vi "TCPPacket Write Body.vi"(8 "error in (no error)":errorcluster, 11 "JSONPacket in":refnum<class "JSONPacket.lvclass">) -> (0 "error out":errorcluster, 2 "Data":u8[](array[numeric]), 3 "JSONPacket out":refnum<class "JSONPacket.lvclass">)   [LabVIEW 2019, in "JSONPacket.lvclass"]
uses:
  JSONPacket.lvclass
  JSONPacket.lvclass/JSONPacket.ctl
  TCPPacket/TCPPacket.lvclass
  <vilib>/addons/Tools/Unicode/UTF8 Tools.lvlib
  6540c986-0add-4175-90d9-41b83a32c240.vi
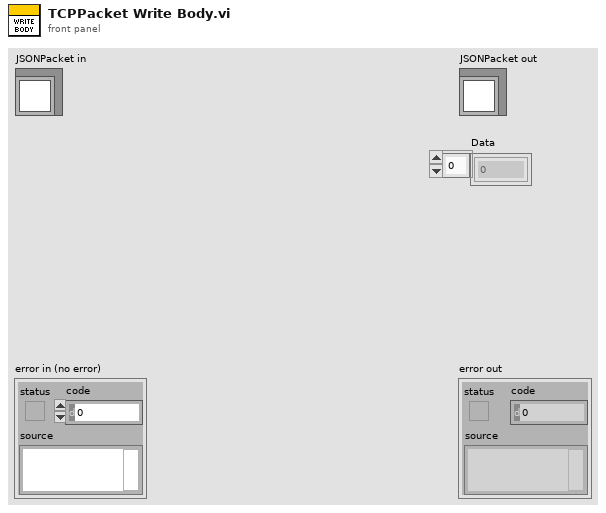
[diagram p1: front panel]
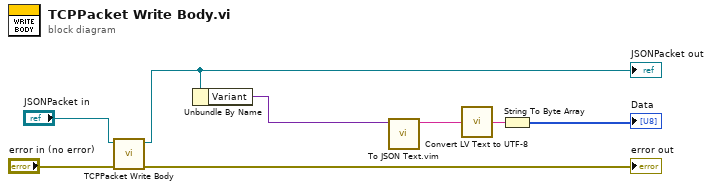
[diagram p0: block diagram]
diagram:
  n1 = call-parent "TCPPacket Write Body.vi"("error in (no error)"="error in (no error)", "TCPPacket in"="JSONPacket in") -> ("error out"=→"error out":errorcluster, "TCPPacket out"=w5:refnum<class "JSONPacket.lvclass">)  [unwired: 7 in, 1 out]
  "JSONPacket out" <- w5
  n2 = Unbundle By Name(w5) -> ("Variant"=w2:variant)
  n3 = call "To JSON Text.vim"("Anything"=w2) -> ("<JSON>"=w1:string)  [unwired: 9 in, 1 out]
  n4 = call <vilib>:"Convert LV Text to UTF-8.vi"("LV Text"=w1) -> ("UTF-8 Text"=w4:string)  [unwired: 13 in, 1 out]
  n5 = String To Byte Array(string=w4) -> (unsigned byte array=→"Data":u8[])
